vi "Rcv Cmd.vi"(8 "error in":errorcluster, 11 "tCRD in":refnum<class "Open Path CRD.lvclass">) -> (0 "error out":errorcluster, 3 "tCRD out":refnum<class "Open Path CRD.lvclass">)   [LabVIEW 2015, in "Open Path CRD.lvclass"]
uses:
  Open Path CRD.lvclass
  Reusable/Instrument/Instrument.lvclass/Instrument.ctl
  Open Path CRD.lvclass/Open Path CRD.ctl
  Reusable/Instrument/state.ctl
  Reusable/Instrument/Read Log Session.vi
  <vilib>/Utility/error.llb/Error Cluster From Error Code.vi
  <vilib>/rvi/errors/niLvFpgaAdjustHostInterfaceError.vi
  Reusable/CRDS/Main/Read Data.vi
  Reusable/CRDS/Data/Main/Read CellData.vi
  Reusable/CRDS/Data/Cell/Read hkParam.vi
  <vilib>/addons/control/pid/pid.llb/PID (DBL).vi
  <userlib>/_Session Fwk/Session - Root.lvclass
  <vilib>/rvi/interface/nirviReadWriteControl/nirviReadWriteControl.xnode
  Open Path FPGA Ref.ctl
  FPGA Bitfiles/80MHz_server.lvbitx
  Reusable/CRDS/Data/Main/CRDS Data.lvclass
  Reusable/CRDS/Data/Cell/CRDS Cell Data.lvclass
  Reusable/Instrument/Instrument.lvclass
  NiFpgaLv.dll
  <vilib>/addons/control/pid/NI_PID_pid.lvlib
  Reusable/Session Log/System Log.lvclass
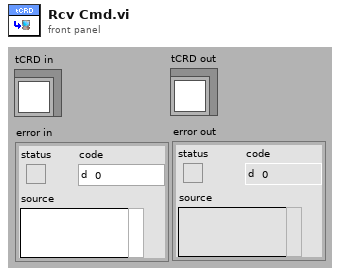
[diagram p1: front panel]
types:
  T1 = typedef "Instrument.lvclass/state.ctl" = enum8{"Configure", "Acquire", "Wait", "Quit", "Handle Error", "NOOP"}
  T2 = typedef "Session - Root.lvclass/Session Handle.ctl" = refnum<data-value>
  T3 = typedef "Open Path CRD.lvclass/Open Path FPGA Ref.ctl" = refnum<k20>
  T4 = cluster{"Array of Double[0]":dbl, "Array of Double[1]":dbl, "Array of Double[2]":dbl}
  T5 = typedef "calData.ctl" = cluster{"rhDilFac":sgl, "Q":sgl, "Tmean":sgl, "extDilFac":sgl, "rhCell":sgl, "P":sgl, "T":sgl}
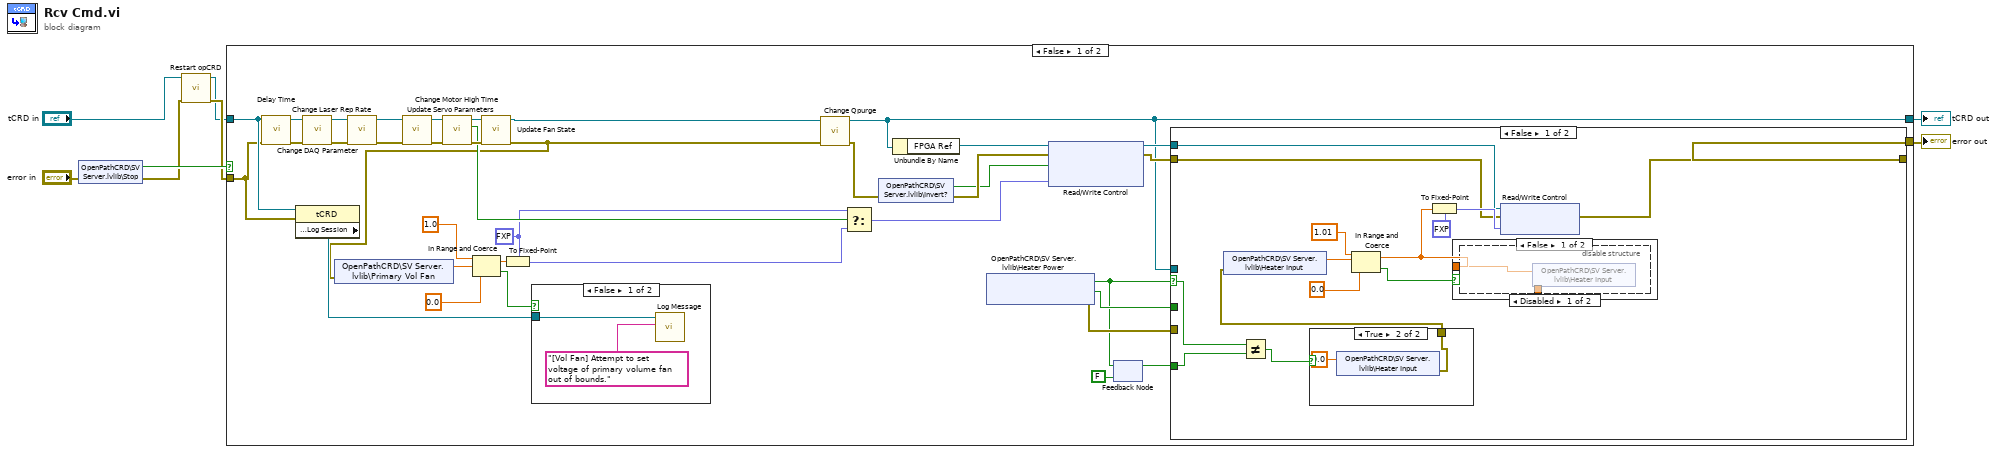
[diagram p0: block diagram]
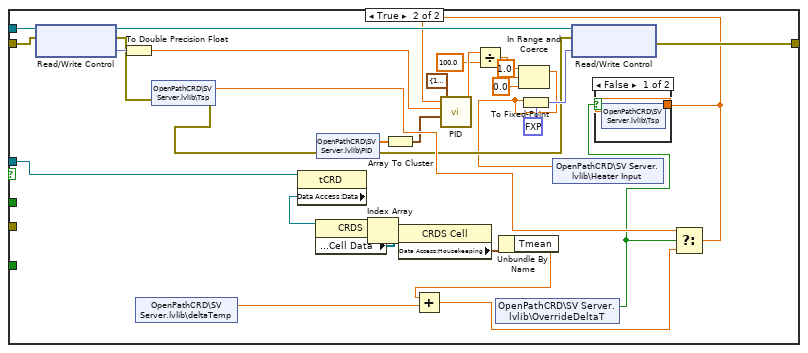
[diagram p6: hidden frame]
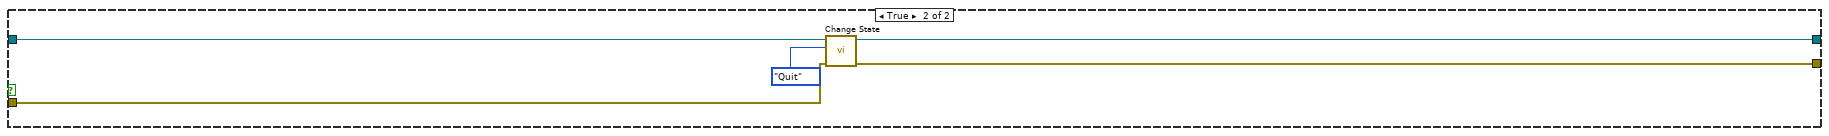
[diagram p8: hidden frame]
diagram:
  n1 = shared-variable "OpenPathCRD\\SV Server.lvlib\\Stop"(error in="error in") -> (w8:bool, error out=w3:errorcluster)
  n2 = call "Restart opCRD.vi"("error in"=w3, "tCRD in"="tCRD in") -> ("error out"=w2:errorcluster, "tCRD out"=w1:refnum<class "Open Path CRD.lvclass">)  [unwired: 8 in]
  n3 = case shown="False" w8 {
    tunnel: w1 -> [w19 w102]
    tunnel: w2 -> [w18 w100]
    tunnel: [w24 w99] -> w6
    tunnel: [w15 w98] -> w5
    frame False {
      w29 = fxp<+/-,20,5> 0.0 ("Primary Vol Fan")
      n4 = call "Delay Time.vi"("error in"=w18, "tCRD in"=w19) -> ("error out"=w44:errorcluster, "tCRD out"=w45:refnum<class "Open Path CRD.lvclass">)  [unwired: 8 in]
      n5 = property class="tCRD"(reference=w19, error in=w18) -> ("Accessors:Log Session"=w16:T2)  [unwired: 2 out]
      n6 = call "Change DAQ Parameter.vi"("error in"=w44, "tCRD in"=w45) -> ("error out"=w41:errorcluster, "tCRD out"=w42:refnum<class "Open Path CRD.lvclass">)  [unwired: 8 in]
      n7 = call "Change Laser Rep Rate.vi"("error in"=w41, "tCRD in"=w42) -> ("error out"=w31:errorcluster, "tCRD out"=w43:refnum<class "Open Path CRD.lvclass">)  [unwired: 8 in]
      n8 = call "Update Servo Parameters.vi"("error in"=w31, "tCRD in"=w43) -> ("error out"=w39:errorcluster, "tCRD out"=w40:refnum<class "Open Path CRD.lvclass">)  [unwired: 8 in]
      n9 = call "Change Motor High Time.vi"("error in"=w39, "tCRD in"=w40) -> ("error out"=w37:errorcluster, "Filter?"=w30:bool, "tCRD out"=w38:refnum<class "Open Path CRD.lvclass">)  [unwired: 7 in]
      n10 = call "Update Fan State.vi"("error in"=w37, "tCRD in"=w38) -> ("error out"=w14:errorcluster, "tCRD out"=w32:refnum<class "Open Path CRD.lvclass">)  [unwired: 8 in]
      n11 = shared-variable "OpenPathCRD\\SV Server.lvlib\\Primary Vol Fan"(error in=w14) -> (w23:dbl)  [unwired: 1 out]
      n12 = In Range and Coerce(upper limit=1.0, x=w23, lower limit=0.0) -> (coerced(x)=w20:dbl, In Range?=w17:bool)
      n13 = To Fixed-Point(fixed-point type=w29, number=w20) -> (fixed-point=w28:fxp<+/-,20,5>)
      n14 = case shown="False" w17 {
        tunnel: w16 -> [w47 _]
        frame False {
          n15 = call "Log Message.vi"("MSG In"="[Vol Fan] Attempt to set voltage of primary volume fan out of bounds.", "session in"=w47) -> ()  [unwired: 8 in, 2 out]
        }
        frame True {
        }
      }
      n16 = call "Change Qpurge.vi"("error in"=w14, "tCRD in"=w32) -> ("error out"=w36:errorcluster, "tCRD out"=w15:refnum<class "Open Path CRD.lvclass">)  [unwired: 8 in]
      n17 = Select(t=w29, s=w30, f=w28) -> (s? t:f=w27:fxp<+/-,20,5>)
      n18 = shared-variable "OpenPathCRD\\SV Server.lvlib\\Invert?"(error in=w36) -> (w33:bool, error out=w34:errorcluster)
      n19 = Unbundle By Name(w15) -> ("FPGA Ref"=w35:T3)
      n20 = shared-variable "OpenPathCRD\\SV Server.lvlib\\Heater Power"() -> (w11:bool, error out=w12:errorcluster, w13:bool)  [unwired: 2 in]
      n21 = xnode "Read/Write Control"("FPGA VI Reference In"=w35, "error in"=w34, "InvertLaser?"=w33, "Primary Vol Fan"=w27) -> ("FPGA VI Reference Out"=w26:T3, "error out"=w25:errorcluster)
      n22 = feedback-in #1(w11) -> ()
      n23 = feedback #1(FALSE ("Boolean")) -> (w9:bool)
      n24 = case shown="False" w11 {
        selector: w11 -> [w50 _]
        tunnel: w26 -> [w59 w96]
        tunnel: w25 -> [w58 w93]
        tunnel: [w57 w90] -> w24
        tunnel: w15 -> [_ w88]
        tunnel: w13 -> [_ _]
        tunnel: w12 -> [_ _]
        tunnel: w9 -> [w51 _]
        frame False {
          n25 = Not Equal?(x=w50, y=w51) -> (x != y?=w49:bool)
          n26 = case shown="True" w49 {
            tunnel: [_ w62] -> w48
            frame False {
            }
            frame True {
              n27 = shared-variable "OpenPathCRD\\SV Server.lvlib\\Heater Input"(0.0 ("Heater Input")) -> (error out=w62:errorcluster)  [unwired: 1 in]
            }
          }
          n28 = shared-variable "OpenPathCRD\\SV Server.lvlib\\Heater Input"(error in=w48) -> (w56:dbl)  [unwired: 1 out]
          n29 = In Range and Coerce(upper limit=1.01, x=w56, lower limit=0.0) -> (coerced(x)=w53:dbl, In Range?=w52:bool)
          n30 = To Fixed-Point(fixed-point type=fxp<+/-,20,5> 0.0 ("Heater Input"), number=w53) -> (fixed-point=w60:fxp<+/-,20,5>)
          n31 = case shown="False" w52 {
            tunnel: w53 -> [w64 _]
            frame False {
              n32 = disable-structure shown="Disabled" {
                disable-tunnel: w64 -> [w65 _]
                frame Disabled {
                  n33 = shared-variable "OpenPathCRD\\SV Server.lvlib\\Heater Input"(w65) -> ()  [unwired: 1 in, 1 out]
                }
                frame Enabled {
                }
              }
            }
            frame True {
            }
          }
          n34 = xnode "Read/Write Control"("FPGA VI Reference In"=w59, "error in"=w58, "Heater Input"=w60) -> ("error out"=w57:errorcluster)  [unwired: 1 out]
        }
        frame True {
          n35 = xnode "Read/Write Control"("FPGA VI Reference In"=w96, "error in"=w93) -> ("FPGA VI Reference Out"=w94:T3, "error out"=w92:errorcluster, "Theatedline"=w95:fxp<+/-,24,12>)
          n36 = To Double Precision Float(number=w95) -> (double precision float=w89:dbl)
          n37 = shared-variable "OpenPathCRD\\SV Server.lvlib\\deltaTemp"() -> (w86:dbl)  [unwired: 1 in, 1 out]
          n38 = shared-variable "OpenPathCRD\\SV Server.lvlib\\Tsp"(error in=w92) -> (w87:dbl, error out=w91:errorcluster)
          n39 = property class="tCRD"(reference=w88) -> ("Data Access:Data"=w73:refnum<class "CRDS Data.lvclass">)  [unwired: 1 in, 2 out]
          n40 = property class="CRDS"(reference=w73) -> ("Data Access:Cell Data"=w72:refnum<class "CRDS Cell Data.lvclass">[])  [unwired: 1 in, 2 out]
          n41 = shared-variable "OpenPathCRD\\SV Server.lvlib\\PID"(error in=w91) -> (w85:dbl[], error out=w80:errorcluster)
          n42 = Index Array(array=w72) -> (element=w71:refnum<class "CRDS Cell Data.lvclass">)  [unwired: 1 in]
          n43 = Array To Cluster(array=w85) -> (cluster=w84:T4)
          n44 = property class="CRDS Cell"(reference=w71) -> ("Data Access:Housekeeping"=w70:T5)  [unwired: 1 in, 2 out]
          n45 = shared-variable "OpenPathCRD\\SV Server.lvlib\\OverrideDeltaT"() -> (w66:bool)  [unwired: 1 in, 1 out]
          n46 = Unbundle By Name(w70) -> ("Tmean"=w69:sgl)
          n47 = Add(x=w69, y=w86) -> (x+y=w68:dbl)
          n48 = Select(t=w87, s=w66, f=w68) -> (s? t:f=w67:dbl)
          n49 = call-poly <vilib>:"PID.vi"("output range"=cluster{"output high":dbl, "output low":dbl} {"output high"=100.0, "output low"=-100.0}, "PID gains"=w84, "process variable"=w89, "setpoint"=w67) -> ("output"=w79:dbl)  [unwired: 6 in, 1 out]
          n50 = Divide(x=w79, y=100.0) -> (x/y=w77:dbl)
          n51 = In Range and Coerce(upper limit=1.0, x=w77, lower limit=0.0) -> (coerced(x)=w74:dbl)  [unwired: 1 out]
          n52 = To Fixed-Point(fixed-point type=fxp<+/-,20,5> 0.0 ("Heater Input"), number=w74) -> (fixed-point=w81:fxp<+/-,20,5>)
          n53 = shared-variable "OpenPathCRD\\SV Server.lvlib\\Heater Input"(w74) -> ()  [unwired: 1 in, 1 out]
          n54 = xnode "Read/Write Control"("FPGA VI Reference In"=w94, "error in"=w80, "Heater Input"=w81) -> ("error out"=w90:errorcluster)  [unwired: 1 out]
          n55 = case shown="False" w66 {
            tunnel: w67 -> [w97 _]
            frame False {
              n56 = shared-variable "OpenPathCRD\\SV Server.lvlib\\Tsp"(w97) -> ()  [unwired: 1 in, 1 out]
            }
            frame True {
            }
          }
        }
      }
    }
    frame True {
      n57 = call "Change State.vi"("error in"=w100, "instr state"=state."Quit", "Instrument in"=w102) -> ("error out"=w99:errorcluster, "Instrument out"=w98:refnum<class "Open Path CRD.lvclass">)  [unwired: 7 in]
    }
  }
  "error out" <- w6
  "tCRD out" <- w5
